vi "Create.vi"(9 "Actor":refnum<class "Actor.lvclass">, 10 "Self Alias":string, 11 "Base Actor in":refnum<class "Base Actor.lvclass">) -> (3 "Base Actor out":refnum<class "Base Actor.lvclass">)   [LabVIEW 2021, in "jettl.lvlib" / "Actor.lvlib" / "Base Actor.lvclass"]
uses:
  Base Actor.lvclass
  Base Actor.lvclass/Base Actor.ctl
  Error/Error.lvlib
  Created Info/Created Info.lvclass
  Addresses Strategy/Addresses Strategy/Addresses Strategy.lvclass
  Actor/Actor.lvclass
  C:/git/jettl/jettl/jettl/Actor/Actor/Actor.lvclass
  C:/git/jettl/jettl/jettl/Last Ack Msg/Last Ack/Last Ack.lvclass
  C:/git/jettl/jettl/jettl/Setup Msg/Setup/Setup.lvclass
  C:/git/jettl/jettl/jettl/Teardown Msg/Teardown/Teardown.lvclass
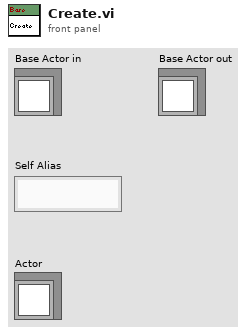
[diagram p1: front panel]
types:
  T1 = typedef "jettl.lvlib/Utilities.lvlib/Created Aliases.ctl" = set{string}
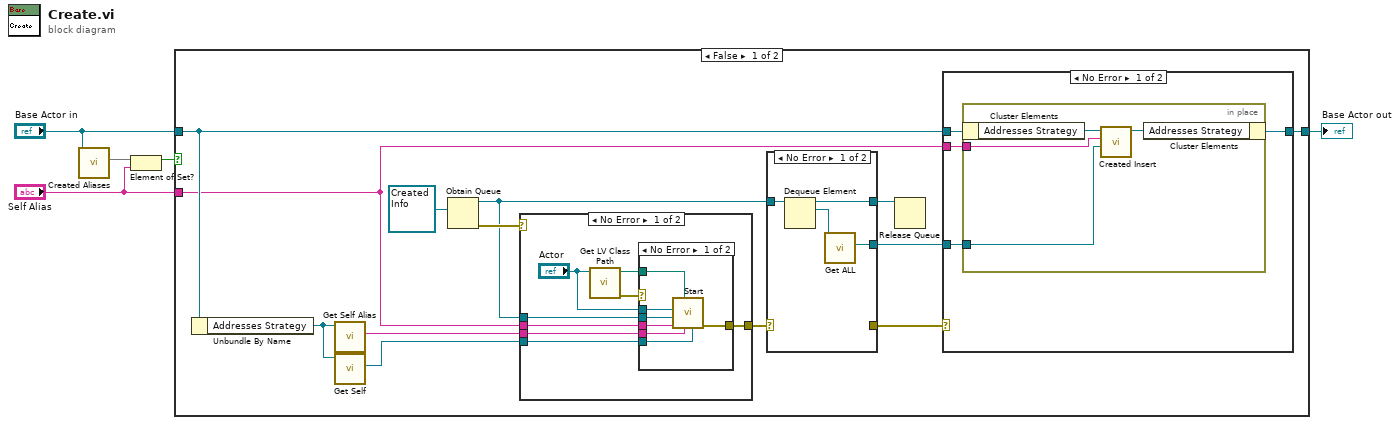
[diagram p0: block diagram]
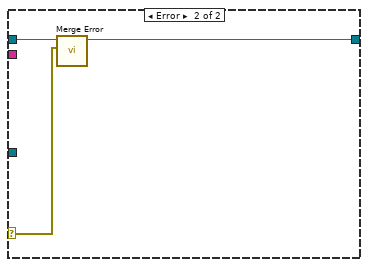
[diagram p5: hidden frame]
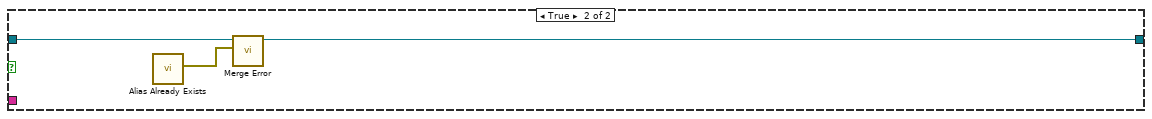
[diagram p6: hidden frame]
diagram:
  n1 = call-dynamic "Created Aliases.vi"("Base Actor in"="Base Actor in") -> ("Created Aliases"=w3:T1)  [unwired: 10 in]
  n2 = Element of Set?(10:"Self Alias", 11:w3) -> (3:w1:bool)
  n3 = case shown="False" w1 {
    tunnel: "Base Actor in" -> [w14 w54]
    tunnel: "Self Alias" -> [w9 _]
    tunnel: [w18 w53] -> w5
    frame False {
      n4 = Unbundle By Name(w14) -> ("Addresses Strategy"=w13:refnum<class "Addresses Strategy.lvclass">)
      n5 = call-dynamic "Get Self Alias.vi"("Addresses Strategy in"=w13) -> ("Self Alias"=w11:string)  [unwired: 10 in]
      n6 = call-dynamic "Get Self.vi"("Addresses Strategy in"=w13) -> ("Self"=w12:refnum<user-event>)  [unwired: 10 in]
      n7 = Obtain Queue(element data type=refnum<class "Created Info.lvclass"> refnum ("jettl.lvlib:Actor.lvlib:Created Info.lvclass")) -> (queue out=w10:refnum<queue>, error out=w17:errorcluster)  [unwired: 4 in, 1 out]
      n8 = case shown="No Error" w17 {
        selector: w17 -> [_ w41]
        tunnel: [w32 w41] -> w15
        tunnel: w9 -> [w29 _]
        tunnel: w12 -> [w31 _]
        tunnel: w11 -> [w30 _]
        tunnel: w10 -> [w28 _]
        frame No Error {
          n9 = call <vilib>:"Get LV Class Path.vi"("object"="Actor") -> ("error out"=w25:errorcluster, "class path"=w26:path)  [unwired: 9 in]
          n10 = case shown="No Error" w25 {
            selector: w25 -> [_ w40]
            tunnel: [w39 w40] -> w32
            tunnel: w31 -> [w38 _]
            tunnel: w30 -> [w37 _]
            tunnel: w29 -> [w36 _]
            tunnel: w28 -> [w33 _]
            tunnel: "Actor" -> [w35 _]
            tunnel: w26 -> [w34 _]
            frame No Error {
              n11 = call "Start.vi"("Creator"=w38, "Creator Alias"=w37, "Path"=w34, "Self Alias"=w36, "Queue of Created Info"=w33, "Actor"=w35) -> ("error out"=w39:errorcluster)  [unwired: 5 in]
            }
            frame Error {
            }
          }
        }
        frame Error {
        }
      }
      n12 = case shown="No Error" w15 {
        selector: w15 -> [_ w24]
        tunnel: [_ w24] -> w16
        tunnel: w10 -> [w22 w23]
        tunnel: [w21 w23] -> w8
        tunnel: [w19 _] -> w7
        frame No Error {
          n13 = Dequeue Element(queue=w22) -> (queue out=w21:refnum<queue>, element=w20:refnum<class "Created Info.lvclass">)  [unwired: 2 in, 2 out]
          n14 = call "Get ALL.vi"("Created Info in"=w20) -> ("Self"=w19:refnum<user-event>)  [unwired: 9 in, 1 out]
        }
        frame Error {
        }
      }
      n15 = Release Queue(queue=w8) -> ()  [unwired: 2 in, 3 out]
      n16 = case shown="No Error" w16 {
        selector: w16 -> [_ w52]
        tunnel: w14 -> [w44 w51]
        tunnel: [w43 w50] -> w18
        tunnel: w9 -> [w45 _]
        tunnel: w7 -> [w42 _]
        frame No Error {
          n17 = in-place {
            in-place-border: w45 -> [w47]
            in-place-border: w42 -> [w46]
            n18 = in-place-cluster #1(w44) -> ("Addresses Strategy"=w49:refnum<class "Addresses Strategy.lvclass">)
            n19 = call-dynamic "Created Insert.vi"("Created"=w46, "Created Alias"=w47, "Addresses Strategy in"=w49) -> ("Addresses Strategy out"=w48:refnum<class "Addresses Strategy.lvclass">)  [unwired: 8 in]
            n20 = in-place-cluster #1("Addresses Strategy"=w48) -> (w43:refnum<class "Base Actor.lvclass">)
          }
        }
        frame Error {
          n21 = call-dynamic "Merge Error.vi"("Error"=w52, "Base Actor in"=w51) -> ("Base Actor out"=w50:refnum<class "Base Actor.lvclass">)  [unwired: 9 in]
        }
      }
    }
    frame True {
      n22 = call "Alias Already Exists.vi"() -> ("Error"=w55:errorcluster)  [unwired: 11 in]
      n23 = call-dynamic "Merge Error.vi"("Error"=w55, "Base Actor in"=w54) -> ("Base Actor out"=w53:refnum<class "Base Actor.lvclass">)  [unwired: 9 in]
    }
  }
  "Base Actor out" <- w5
